vi "json approval test.vi"() -> ()   [LabVIEW 2020]
uses:
  Person/Person.lvclass
  <vilib>/PNR/JSONtext Object Serialization/Generic Object Serializer/Generic Object Serializer.lvclass
  C:/Program Files/National Instruments/LabVIEW 2020/vi.lib/JDP Science/JSONtext/LVClass Serializer/JSONtext LVClass Serializer.lvclass
  Person/Person.lvclass/Person.ctl
  29ce0495-dfe1-4fb6-a024-e9bbcee7fb6c.vi
  Person/Write First Name.vi
  Person/Write Last Name.vi
  Person/Write Title.vi
  <vilib>/JDP Science/JSONtext/Variant to JSON Text.vi
  <vilib>/addons/_JKI Toolkits/Caraya/classes/Assert/Assert True.vi
  <vilib>/addons/_JKI Toolkits/Caraya/classes/Test/Test.lvclass
  <vilib>/addons/_JKI Toolkits/Caraya/classes/Assert/Assert.lvclass
  Approval Tests/Approval Tests.lvlib
panel:
  out "Failure Message":string
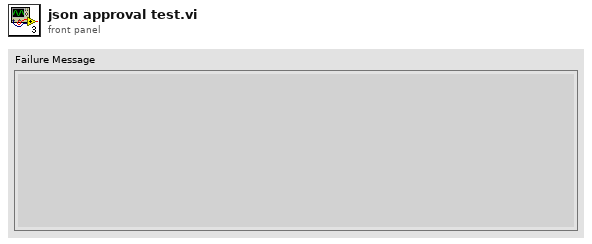
[diagram p1: front panel]
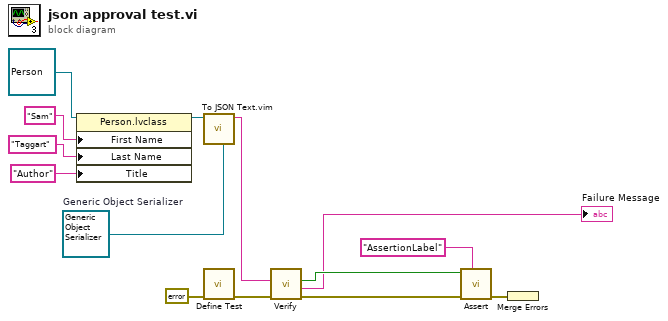
[diagram p0: block diagram]
diagram:
  w1 = refnum<class "Generic Object Serializer.lvclass"> refnum  # Generic Object Serializer
  n1 = property on="Property Node" class="Person.lvclass"(reference=refnum<class "Person.lvclass"> refnum ("Person.lvclass"), "First Name"="Sam" ("Test Data"), "Last Name"="Taggart" ("Test Data"), "Title"="Author" ("Test Data")) -> (reference out=w2:refnum<class "Person.lvclass">)  [unwired: 1 in, 1 out]
  n2 = call "To JSON Text.vim"("LVClass Serializer"=w1, "Anything"=w2) -> ("<JSON>"=w3:string)  [unwired: 8 in, 1 out]
  n3 = call <vilib>:"Define Test.vi"("error in (no error)"=errorcluster {"status"=FALSE, "code"=0, "source"=""}) -> ("error out"=w11:errorcluster)  [unwired: 9 in, 1 out]
  n4 = call "Verify.vi"("error in"=w11, "Test Data"=w3) -> ("error out"=w10:errorcluster, "Failure Message"=→"Failure Message":string, "Passed?"=w9:bool)  [unwired: 7 in]
  n5 = call-poly <vilib>:"Assert.vi"("Label"="AssertionLabel" ("Label (VI Title)"), "error in (no error)"=w10, "True?"=w9) -> ("error out"=w13:errorcluster)  [unwired: 7 in, 1 out]
  n6 = Merge Errors(w13) -> ()  [unwired: 1 out]
